vi "CenterX.vi"() -> ()   [LabVIEW 2015]
panel:
  out "CenterX":dbl
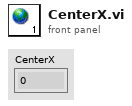
[diagram p1: front panel]
diagram:
